vi "Z Aux Search Eth.vi"(8 "error in (no error)":errorcluster caption="错误输入（无错误）", 10 "uims":u32, 11 "ipaddress":string) -> (0 "error out":errorcluster caption="错误输出", 3 "function return":i32)   [LabVIEW 2015, in "zauxdll.lvlib"]
doc: "int32 __stdcall ZAux_SearchEth(const char *ipaddress, uint32 uims);"
uses:
  zauxdll.lvlib
  Radar - 2015 32bit_autoqueue_angle_0319/zauxdll-2014/zauxdll.dll
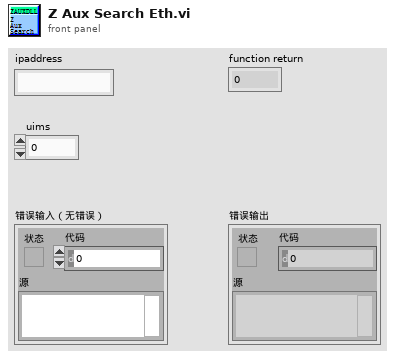
[diagram p1: front panel]
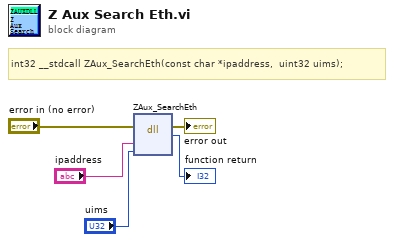
[diagram p0: block diagram]
diagram:
  # "int32 __stdcall ZAux_SearchEth(const char *ipaddress,  uint32 uims);"
  n1 = dll-call lib="D:/vicomm case/cub/0717/Radar - 2015 32bit_autoqueue_angle_0319/zauxdll-2014/zauxdll.*" fn="ZAux_SearchEth"(error in="error in (no error)", "ipaddress"="ipaddress", "uims"="uims") -> (error out=→"error out":errorcluster, →"function return":i32)  [unwired: 4 in, 1 out]
